vi "Alarm (SubVI).vi"(9 "String":string, 10 "Elapsed Time":timestamp, 11 "Byte Stream File in":refnum<file>) -> (3 "Alarm Indicator":bool)   [LabVIEW 2013]
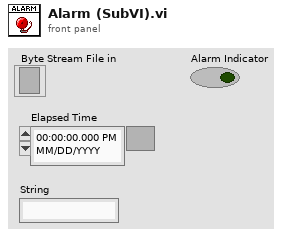
[diagram p1: front panel]
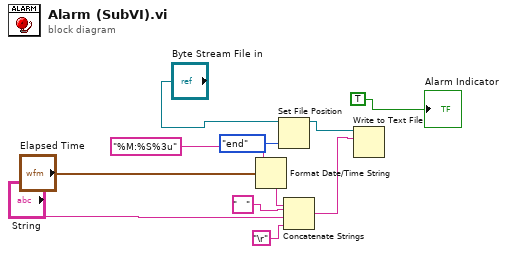
[diagram p0: block diagram]
diagram:
  n1 = Format Date/Time String(time format string (%c)="%M:%S%3u", seconds (now)="Elapsed Time") -> (date/time string=w10:string)  [unwired: 1 in]
  n2 = Set File Position(refnum="Byte Stream File in", from (0:start)=enum16{"start", "end", "current"}."end") -> (refnum out=w4:refnum<file>)  [unwired: 2 in, 1 out]
  n3 = Concatenate Strings(w10, "   " ("string"), "String", "\r") -> (w5:string)
  n4 = Write to Text File(file (use dialog)=w4, text=w5) -> ()  [unwired: 2 in, 3 out]
  "Alarm Indicator" <- TRUE ("1201")
